vi "exclude.get.vi"(8 "error in (no error)":errorcluster, 11 "exclude in":refnum<class "exclude.lvclass">) -> (0 "error out":errorcluster, 2 "exclude":set{refnum<class "filterTypes.lvclass">}(c389), 3 "exclude out":refnum<class "exclude.lvclass">)   [LabVIEW 2020, in "nominal types.lvlib" / "channelFilter.lvlib" / "exclude.lvclass"]
uses:
  exclude.lvclass
  exclude.lvclass/exclude.ctl
  filterTypes/filterTypes.lvclass
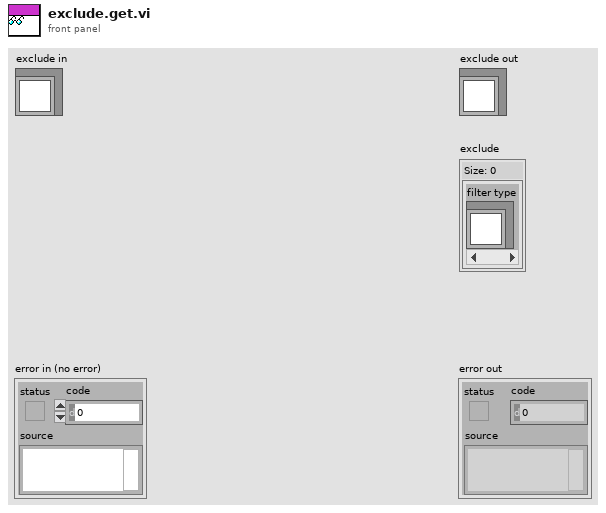
[diagram p1: front panel]
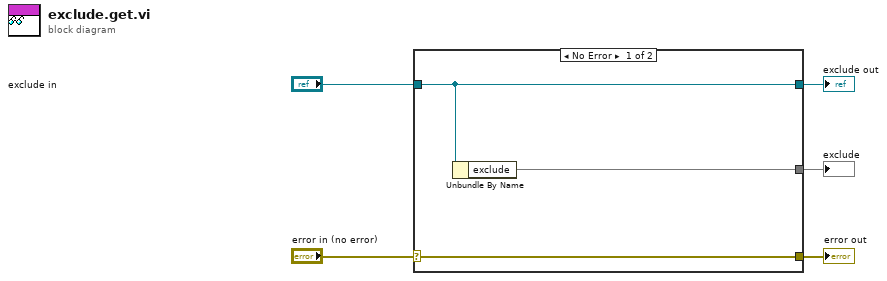
[diagram p0: block diagram]
diagram:
  n1 = case shown="No Error" "error in (no error)" {
    selector: "error in (no error)" -> [w8 w9]
    tunnel: [w8 w9] -> w4
    tunnel: [w7 w10] -> w2
    tunnel: "exclude in" -> [w7 w10]
    tunnel: [w6 _] -> w1
    frame No Error {
      n2 = Unbundle By Name(w7) -> ("exclude"=w6:set{refnum<class "filterTypes.lvclass">})
    }
    frame Error {
    }
  }
  "error out" <- w4
  "exclude out" <- w2
  "exclude" <- w1
